vi "New GPS on GIC C.vi"(11 "GIC Input":T1={"     Use ?\nOff       On"=[FALSE, TRUE, FALSE, TRUE], "Mode:"=FALSE, "Extra Port"="", "Hokuyo Port"="COM7", "Tx Prop  Port"="COM6", "Compass Port"="", "GPS Port"="", "Num of WPs"=0, "WP Lats and Longs"={"WP Lats"=[], "WP Longs"=[]}, "Obst Lats and Longs"={"Obst Lats"=[], "Obst Longs"=[]}, "Parameters"=[], "GPS Data"=[], "Compass"=0.0, "LMS Vector"=[], "Vision Vector"=[], "Direction Cmd"=0.0, "Speed Cmd"=0.0, "WP Vector"=[], "WP Number"=0, "Extra"=0, "SW Map"=[], "Path Cluster"={"Path x node"=[], "Path y node"=[]}, "Sim Course"=[]} {"Obst Lats and Longs"."Obst Longs" format="%#_8g"; "Obst Lats and Longs"."Obst Lats" format="%#_8g"}) -> (3 "GIC Output":T1={"     Use ?\nOff       On"=[FALSE, TRUE, FALSE, TRUE], "Mode:"=FALSE, "Extra Port"="", "Hokuyo Port"="COM7", "Tx Prop  Port"="COM6", "Compass Port"="", "GPS Port"="", "Num of WPs"=0, "WP Lats and Longs"={"WP Lats"=[], "WP Longs"=[]}, "Obst Lats and Longs"={"Obst Lats"=[], "Obst Longs"=[]}, "Parameters"=[], "GPS Data"=[], "Compass"=0.0, "LMS Vector"=[], "Vision Vector"=[], "Direction Cmd"=0.0, "Speed Cmd"=0.0, "WP Vector"=[], "WP Number"=0, "Extra"=0, "SW Map"=[], "Path Cluster"={"Path x node"=[], "Path y node"=[]}, "Sim Course"=[]} {"Obst Lats and Longs"."Obst Longs" format="%#_8g"; "Obst Lats and Longs"."Obst Lats" format="%#_8g"})   [LabVIEW 2014]
panel:
  # "New GPS on GIC C"
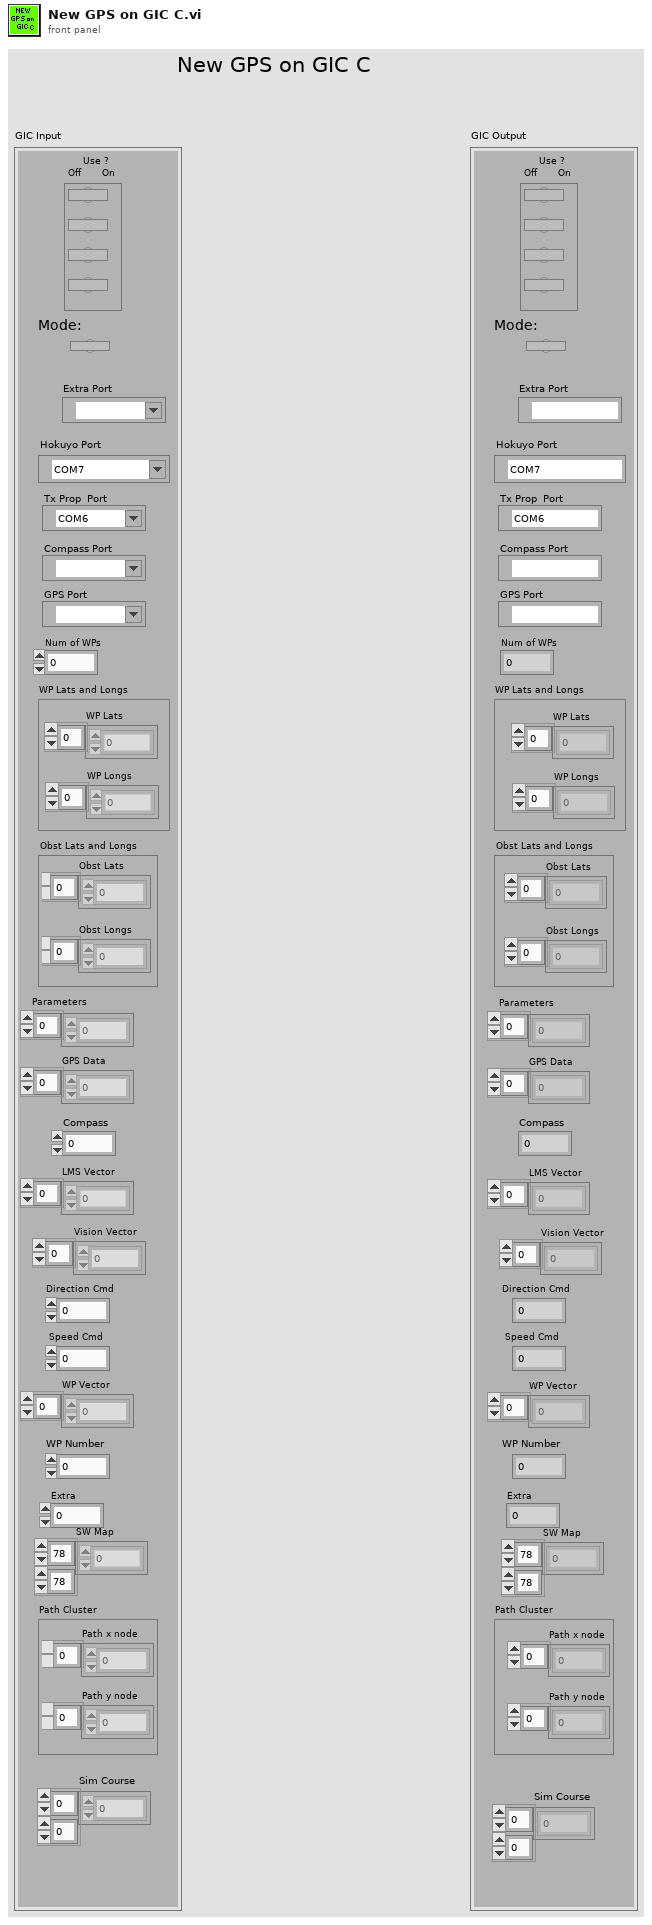
[diagram p1: front panel]
types:
  T1 = cluster{"     Use ?\nOff       On":bool[], "Mode:":bool, "Extra Port":refnum<visa-resource-name>, "Hokuyo Port":refnum<visa-resource-name>, "Tx Prop  Port":refnum<visa-resource-name>, "Compass Port":refnum<visa-resource-name>, "GPS Port":refnum<visa-resource-name>, "Num of WPs":i16, "WP Lats and Longs":cluster{"WP Lats":dbl[], "WP Longs":dbl[]}, "Obst Lats and Longs":cluster{"Obst Lats":dbl[], "Obst Longs":dbl[]}, "Parameters":dbl[], "GPS Data":dbl[], "Compass":dbl, "LMS Vector":dbl[], "Vision Vector":dbl[], "Direction Cmd":dbl, "Speed Cmd":dbl, "WP Vector":dbl[], "WP Number":i32, "Extra":i16, "SW Map":i32[][], "Path Cluster":cluster{"Path x node":dbl[], "Path y node":dbl[]}, "Sim Course":i8[][]}
  T2 = cluster{"     Use ?\nOff       On":bool[], "Mode:":bool, "Rx Prop Port":refnum<visa-resource-name>, "Hokuyo Port":refnum<visa-resource-name>, "Tx Prop  Port":refnum<visa-resource-name>, "Compass Port":refnum<visa-resource-name>, "GPS Port":refnum<visa-resource-name>, "Num of WPs":i16, "WP Lats and Longs":cluster{"WP Lats":dbl[], "WP Longs":dbl[]}, "Obst Lats and Longs":cluster{"Obst Lats":dbl[], "Obst Longs":dbl[]}, "Parameters":dbl[], "GPS Data":dbl[], "Compass":dbl, "LMS Vector":dbl[], "Vision Vector":dbl[], "Direction Cmd":dbl, "Speed Cmd":dbl, "WP Vector":dbl[], "WP Number":i32, "Extra":i16, "SW Map":i32[][], "Path Cluster":cluster{"Path x node":dbl[], "Path y node":dbl[]}, "Sim Course":i8[][]}
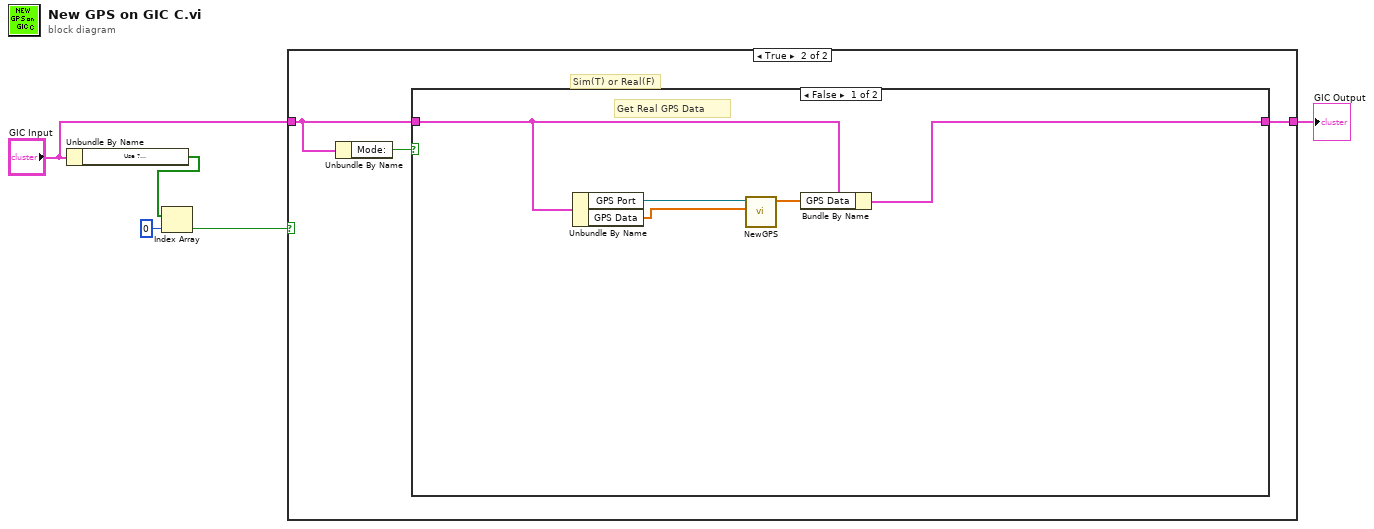
[diagram p0: block diagram]
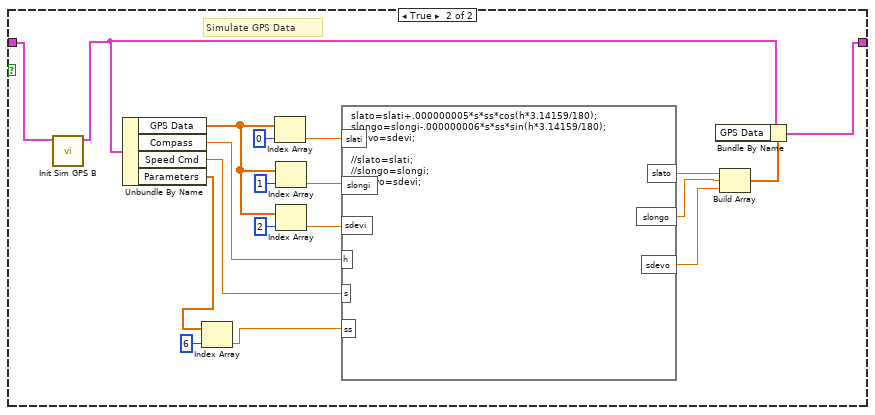
[diagram p3: hidden frame]
diagram:
  n1 = Unbundle By Name("GIC Input") -> ("Use ?\nOff       On"=w5:bool[])
  n2 = Index Array(array=w5, index=0) -> (element=w3:bool)
  n3 = case shown="True" w3 {
    tunnel: "GIC Input" -> [w6 w8]
    tunnel: [w6 w7] -> w1
    frame False {
    }
    frame True {
      # "Sim(T) or Real(F)"
      n4 = Unbundle By Name(w8) -> ("Mode:"=w9:bool)
      n5 = case shown="False" w9 {
        tunnel: w8 -> [w12 w19]
        tunnel: [w10 w20] -> w7
        frame False {
          # "Get Real GPS Data"
          n6 = Unbundle By Name(w12) -> ("GPS Port"=w14:refnum<visa-resource-name>, "GPS Data"=w13:dbl[])
          n7 = call "NewGPS.vi"("Input lat, long, dev"=w13, "GPS Com Port"=w14) -> ("Output lat, long, dev"=w11:dbl[])  [unwired: 9 in]
          n8 = Bundle By Name(cluster=w12, "GPS Data"=w11) -> (w10:T1)
        }
        frame True {
          # "Simulate GPS Data"
          n9 = call "Init Sim GPS B.vi"("GIC Input"=w19) -> ("GIC Output"=w18:T2)  [unwired: 10 in]
          n10 = Unbundle By Name(w18) -> ("GPS Data"=w29:dbl[], "Compass"=w26:dbl, "Speed Cmd"=w25:dbl, "Parameters"=w17:dbl[])
          n11 = Index Array(array=w17, index=6) -> (element=w15:dbl)
          n12 = Index Array(array=w29, index=0) -> (element=w33:dbl)
          n13 = Index Array(array=w29, index=1) -> (element=w31:dbl)
          n14 = Index Array(array=w29, index=2) -> (element=w28:dbl)
          n15 = formula code="slato=slati+.000000005*s*ss*cos(h*3.14159/180);\nslongo=slongi-.000000006*s*ss*sin(h*3.14159/180);\nsdevo=sdevi;\n\n//slato=slati;\n//slongo=slongi;\n//sdevo=sdevi;"("slati"=w33, "slongi"=w31, "sdevi"=w28, "h"=w26, "s"=w25, "ss"=w15) -> ("slato"=w24:dbl, "slongo"=w23:dbl, "sdevo"=w22:dbl)
          n16 = Build Array(w24, w23, w22) -> (w21:dbl[])
          n17 = Bundle By Name(cluster=w18, "GPS Data"=w21) -> (w20:T2)
        }
      }
    }
  }
  "GIC Output" <- w1
